vi "XceiverCmds.vi"(0 "RF Chip0 Channel":u8, 1 "RF Chip0 Enable":bool, 3 "RF Chip1 Enable":bool, 5 "RF Chip1 Channel":u8, 7 "DUT Serial #":i32, 9 "mSec":u8, 11 "error in (no error)":errorcluster, 12 "XceiverCmd":T1=enum."Load&Xmit") -> (4 "unsigned byte array":u8[](array[numeric]) format="%x", 6 "RF Channel Out":u8, 15 "error out":errorcluster)   [LabVIEW 2015]
uses:
  XceiverCmds.ctl
  XceiverStates.ctl
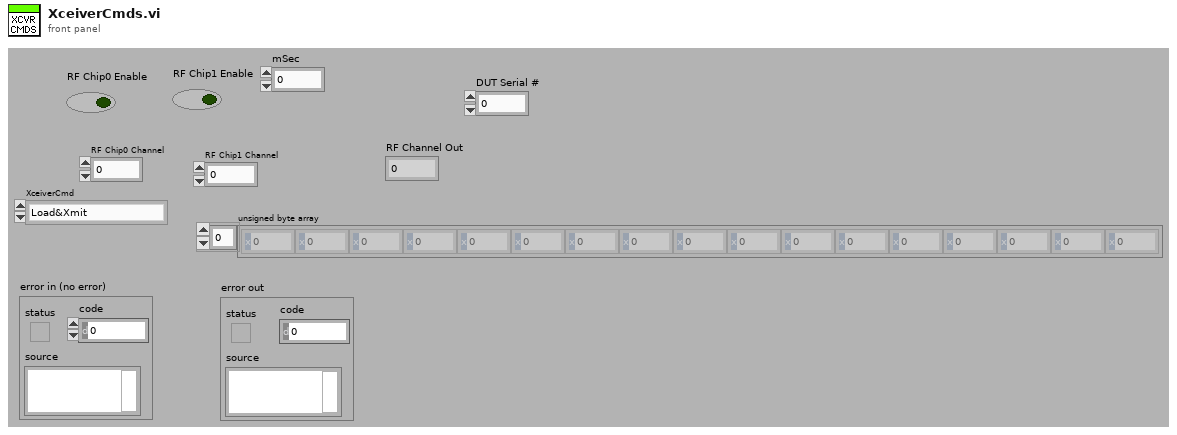
[diagram p1: front panel]
types:
  T1 = typedef "XceiverCmds.ctl" = enum8{"Get Window", "Set Window", "Load&Xmit", "Find Window", "Load CC1101", "Blink LED1", "Blink LED2", "Gen2 Mode", "Request Rev", "Gen2 Mode & Req Rev", "Load Device Settings", "Reset Xceiver", "Set Channel", "Read Channel"}
  T2 = typedef "XceiverStates.ctl" = enum16{"Initialize", "Rx", "Tx", "Raw Mode", "Clear Buffer", "ClearEcho", "Read Buffer", "Close"}
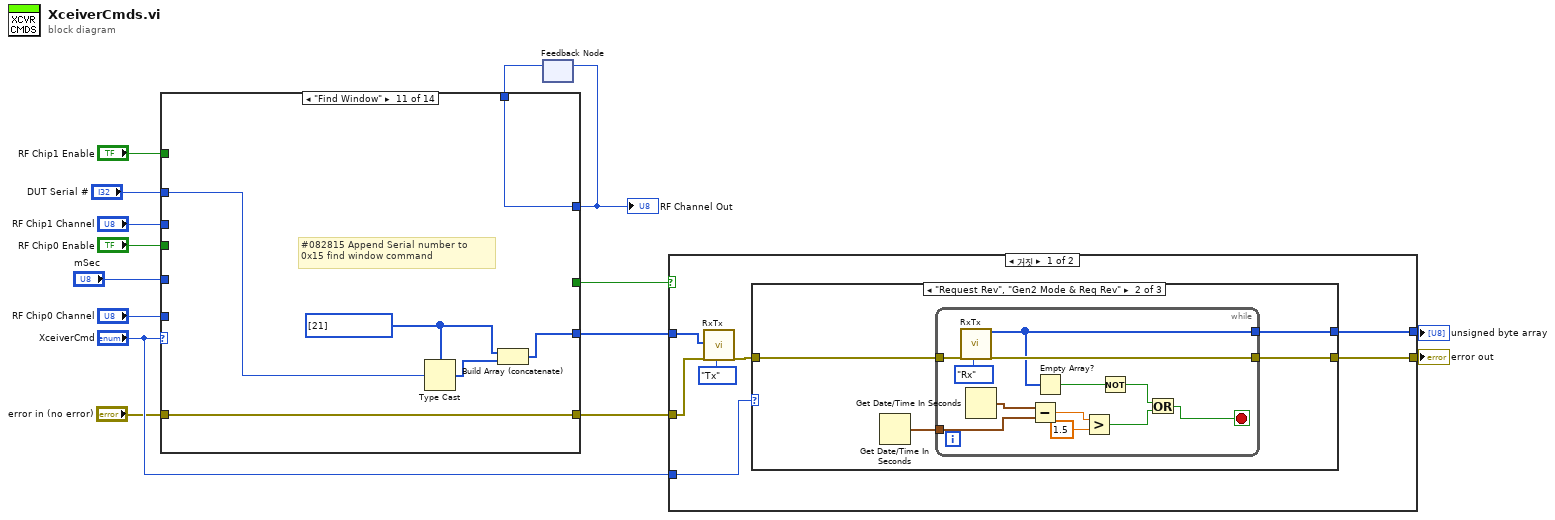
[diagram p0: block diagram]
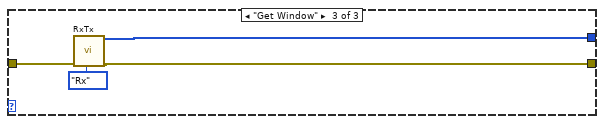
[diagram p3: hidden frame]
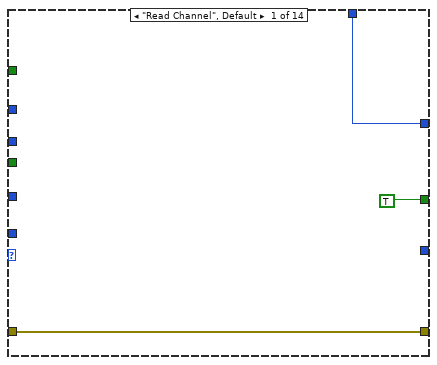
[diagram p5: hidden frame]
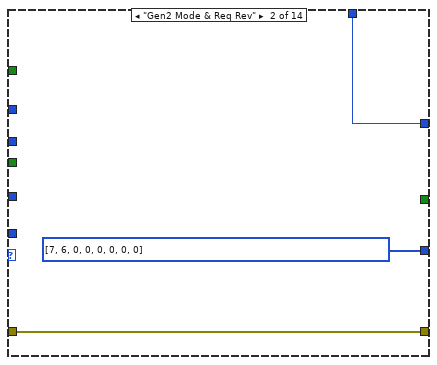
[diagram p6: hidden frame]
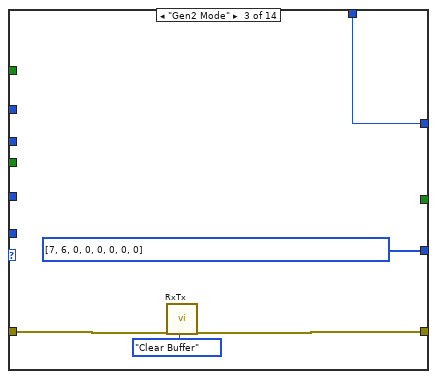
[diagram p7: hidden frame]
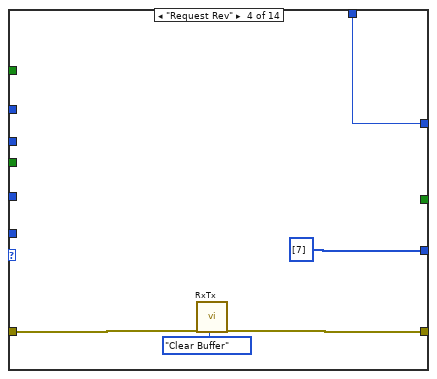
[diagram p8: hidden frame]
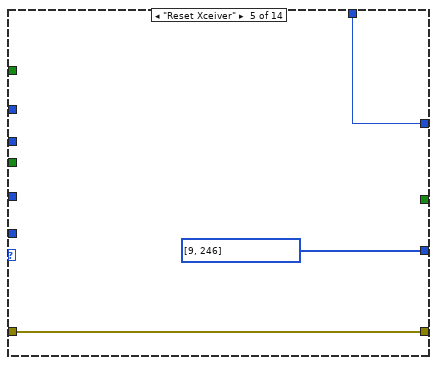
[diagram p9: hidden frame]
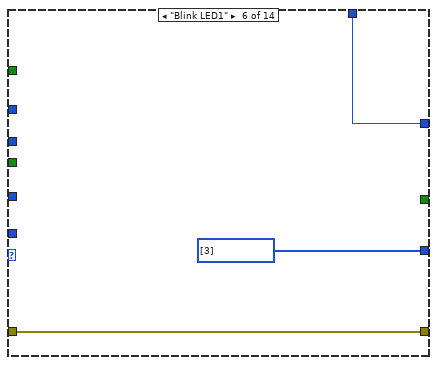
[diagram p10: hidden frame]
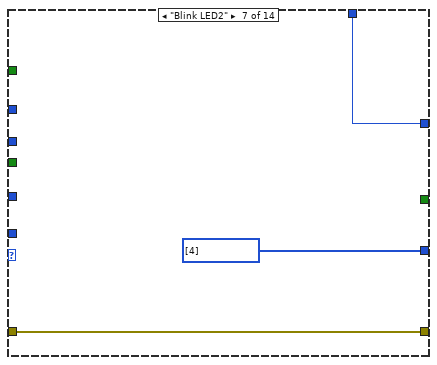
[diagram p11: hidden frame]
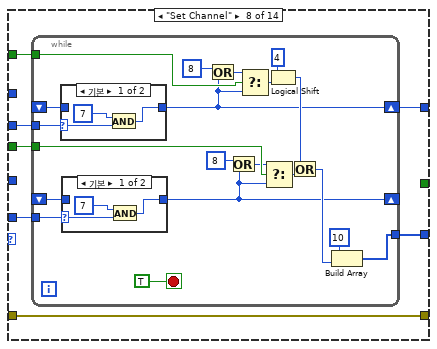
[diagram p12: hidden frame]
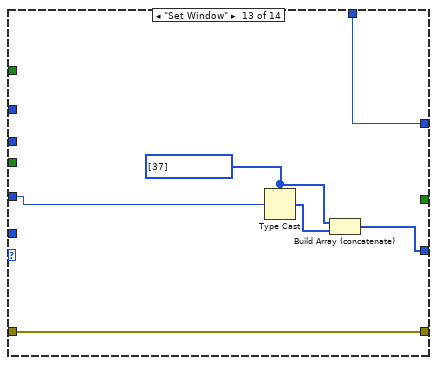
[diagram p18: hidden frame]
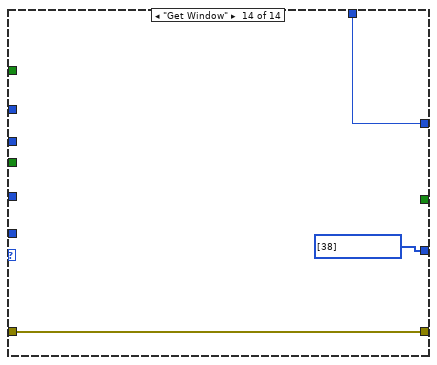
[diagram p19: hidden frame]
diagram:
  n1 = feedback #1() -> (w3:u8)  [unwired: 1 in]
  n2 = case shown="\"Find Window\"" "XceiverCmd" {
    tunnel: [_ u8[] [7, 6, 0, 0, 0, 0, 0, 0] u8[] [7, 6, 0, 0, 0, 0, 0, 0] u8[] [7] u8[] [9, 246] u8[] [3] u8[] [4] w47 _ _ w80 _ w88 u8[] [38]] -> w6
    tunnel: "error in (no error)" -> [w18 w19 w24 w29 w33 w37 w40 w46 w77 w79 w85 w87 w93 w96]
    tunnel: [w18 w19 w23 w28 w33 w37 w40 w46 w77 w79 w85 w87 w93 w96] -> w12
    tunnel: "RF Chip0 Channel" -> [_ _ _ _ _ _ _ w42 _ _ _ _ _ _]
    tunnel: "RF Chip1 Channel" -> [_ _ _ _ _ _ _ w45 _ _ _ _ _ _]
    tunnel: "RF Chip1 Enable" -> [_ _ _ _ _ _ _ w44 _ _ _ _ _ _]
    tunnel: "RF Chip0 Enable" -> [_ _ _ _ _ _ _ w43 _ _ _ _ _ _]
    tunnel: [TRUE _ _ _ _ _ _ _ _ _ _ _ _ _] -> w5
    tunnel: [w16 w20 w22 w27 w32 w35 w38 w41 w76 w78 w84 w86 w92 w95] -> w4
    tunnel: w3 -> [w16 w20 w22 w27 w32 w35 w38 _ w76 w78 w84 w86 w92 w95]
    tunnel: "mSec" -> [_ _ _ _ _ _ _ _ _ _ _ _ w91 _]
    tunnel: "DUT Serial #" -> [_ _ _ _ _ _ _ _ _ _ w82 _ _ _]
    frame "Read Channel", Default {
    }
    frame "Gen2 Mode & Req Rev" {
    }
    frame "Gen2 Mode" {
      n3 = call "RxTx.vi"("error in (no error)"=w24, "Action"=XceiverStates."Clear Buffer") -> ("error out"=w23:errorcluster)  [unwired: 9 in, 8 out]
    }
    frame "Request Rev" {
      n4 = call "RxTx.vi"("error in (no error)"=w29, "Action"=XceiverStates."Clear Buffer") -> ("error out"=w28:errorcluster)  [unwired: 9 in, 8 out]
    }
    frame "Reset Xceiver" {
    }
    frame "Blink LED1" {
    }
    frame "Blink LED2" {
    }
    frame "Set Channel" {
      n5 = while {
        tunnel: [w67] -> w47
        tunnel: w45 -> [w65]
        shift-right: [w50] -> w41
        shift-left: _ -> [w64]
        tunnel: w44 -> [w62]
        tunnel: w42 -> [w57]
        shift-right: [w49] -> _
        shift-left: _ -> [w58]
        tunnel: w43 -> [w61]
        stop <- TRUE stop-if-true
        n6 = case shown="기본" w65 {
          selector: w65 -> [w74 _]
          tunnel: [w73 w75] -> w50
          tunnel: w64 -> [_ w75]
          frame Default {
            n7 = And(x=u8 7, y=w74) -> (x .and. y?=w73:u8)
          }
          frame 0 {
          }
        }
        n8 = case shown="기본" w57 {
          selector: w57 -> [w70 _]
          tunnel: [w69 w71] -> w49
          tunnel: w58 -> [_ w71]
          frame Default {
            n9 = And(x=u8 7, y=w70) -> (x .and. y?=w69:u8)
          }
          frame 0 {
          }
        }
        n10 = Or(x=u8 8, y=w50) -> (x .or. y?=w63:u8)
        n11 = Or(x=u8 8, y=w49) -> (x .or. y?=w60:u8)
        n12 = Select(t=w63, s=w62, f=w50) -> (s? t:f=w54:u8)
        n13 = Select(t=w60, s=w61, f=w49) -> (s? t:f=w55:u8)
        n14 = Logical Shift(y=i8 4, x=w54) -> (x << y=w53:u8)
        n15 = Or(x=w53, y=w55) -> (x .or. y?=w66:u8)
        n16 = Build Array(u8 10, w66) -> (w67:u8[])
      }
    }
    frame "Load Device Settings" {
    }
    frame "Load CC1101" {
    }
    frame "Find Window" {
      w83 = u8[] [21]
      # "#082815 Append Serial number to \n0x15 find window command"
      n17 = Type Cast(type=w83, x=w82) -> (*(type *) &x=w81:u8[])
      n18 = Build Array (concatenate)(w83, w81) -> (w80:u8[])
    }
    frame "Load&Xmit" {
    }
    frame "Set Window" {
      w90 = u8[] [37]
      n19 = Type Cast(type=w90, x=w91) -> (*(type *) &x=w89:u8[])
      n20 = Build Array (concatenate)(w90, w89) -> (w88:u8[])
    }
    frame "Get Window" {
    }
  }
  "RF Channel Out" <- w4
  n21 = feedback-in #1(w4) -> ()
  n22 = case shown="거짓" w5 {
    tunnel: [w102 w125] -> w15
    tunnel: "XceiverCmd" -> [w101 _]
    tunnel: w12 -> [w100 w125]
    tunnel: [w99 w126] -> w11
    tunnel: w6 -> [w97 w126]
    frame False {
      n23 = call "RxTx.vi"("[TxData]"=w97, "error in (no error)"=w100, "Action"=XceiverStates."Tx") -> ("error out"=w103:errorcluster)  [unwired: 8 in, 8 out]
      n24 = case shown="\"Request Rev\", \"Gen2 Mode & Req Rev\"" w101 {
        tunnel: w103 -> [w104 w108 w123]
        tunnel: [w104 w107 w122] -> w102
        tunnel: [_ w106 w121] -> w99
        frame "Load&Xmit", Default {
        }
        frame "Request Rev", "Gen2 Mode & Req Rev" {
          n25 = Get Date/Time In Seconds() -> (seconds since 1Jan1904=w105:timestamp)
          n26 = while {
            tunnel: w108 -> [w120]
            tunnel: [w119] -> w107
            tunnel: [w117] -> w106
            tunnel: w105 -> [w109]
            stop <- w111 stop-if-true
            n27 = call "RxTx.vi"("error in (no error)"=w120, "Action"=XceiverStates."Rx") -> ("[Raw RxData]"=w117:u8[], "error out"=w119:errorcluster)  [unwired: 9 in, 7 out]
            n28 = Get Date/Time In Seconds() -> (seconds since 1Jan1904=w110:timestamp)
            n29 = Subtract(x=w110, y=w109) -> (x-y=w115:dbl)
            n30 = Empty Array?(array=w117) -> (empty?=w116:bool)
            n31 = Greater?(x=w115, y=1.5) -> (0:w112:bool)
            n32 = Not(x=w116) -> (.not. x?=w113:bool)
            n33 = Or(x=w113, y=w112) -> (x .or. y?=w111:bool)
          }
        }
        frame "Get Window" {
          n34 = call "RxTx.vi"("error in (no error)"=w123, "Action"=XceiverStates."Rx") -> ("[Raw RxData]"=w121:u8[], "error out"=w122:errorcluster)  [unwired: 9 in, 7 out]
        }
      }
    }
    frame True {
    }
  }
  "error out" <- w15
  "unsigned byte array" <- w11
